vi "niFpgaMemoryEmulationRefIn.vi"(0 "Address":u32, 1 "Name":variant, 5 "Data":i32, 7 "Write? (F)":bool, 9 "inTimedLoop":bool, 11 "error in (no error)":errorcluster, 12 "Node Link":cluster{"VIRef":refnum<vi>, "UID":i32}) -> (6 "Data":i32, 15 "error out":errorcluster)   [LabVIEW 2017]
uses:
  <vilib>/rvi/DataTransferAndStorage/Container/Common/niFpgaContainerMetaDataKey.ctl
  <instcachedir>/0/nirvimemoryFastEmulation_424FDD443BC54103A00327FF1F2580B8.lvgen/nirvimemoryFastEmulation_424FDD443BC54103A00327FF1F2580B8_000.vi
  <instcachedir>/0/nirvimemoryEmulation_DE953D9D328548638838B08CDB120B27.lvgen/nirvimemoryEmulation_DE953D9D328548638838B08CDB120B27_000.vi
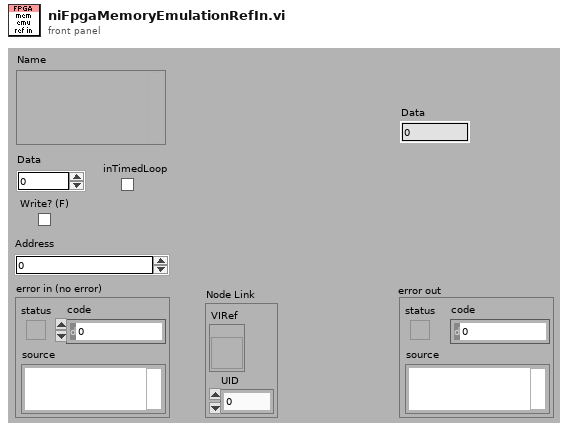
[diagram p1: front panel]
types:
  T1 = typedef "niFpgaContainerMetaDataKey.ctl" = enum16{"FPGA FIFO", "FPGA Memory", "FPGA Register", "FPGA Handshake"}
  T2 = typedef "niFpgaContainerState.ctl" = cluster{"displayName":string, "hardwareName":string, "dataType":T3, "elementTypeDescriptor":variant, "terminalTypeDescriptor":variant, "requestedNumberOfElements":u32, "memoryType":T4, "arbitrationForInterfaceA":T5, "numberOfElementsPerRead":u32, "arbitrationForInterfaceB":T5, "numberOfElementsPerWrite":u32, "VI_Defined":bool, "type":T6, "initializationParameters":T7, "disableOnOverflow/Underflow":bool, "interfaceConfiguration":T8, "controlLogic":T9, "actualNumberOfElements":u32, "dramSelection":string, "dramMaxOustandingRequests":i32, "dramIncludeByteEnables":bool, "dramGrantTime":u32, "fullEmulation":bool, "memoryInMultipleClockDomains":bool, "memoryLatency":T10}
  T3 = typedef "niFpgaDataTypeControl.ctl" = enum32{"Boolean", "I8", "I16", "I32", "I64", "U8", "U16", "U32", "U64", "FXP", "CustomControl", "SGL"}
  T4 = typedef "niFpgaContainerImplementationControl.ctl" = enum16{"Flip-Flops", "Look-Up Table", "Block Memory", "DRAM"}
  T5 = typedef "niFpgaContainerArbitrationOptionsControl.ctl" = enum16{"Always Arbitrate", "Arbitrate if Multiple Requestors Only", "Never Arbitrate"}
  T6 = typedef "niFpgaTransferTypeControl.ctl" = enum16{"Target-Scoped", "Host to Target - DMA", "Target to Host - DMA", "Peer to Peer Reader", "Peer to Peer Writer", "Bidirectional"}
  T7 = typedef "niFpgaContainerInitializationParameters.ctl" = cluster{"initialized":bool, "VI_Path":path, "initialData":variant}
  T8 = typedef "niFpgaMemoryInterfaceConfiguration.ctl" = enum16{"Read A-Write B", "Read A-Read B"}
  T9 = typedef "niFpgaFifoControlLogicControl.ctl" = enum16{"Slice Fabric", "Target Optimal", "Built-in"}
  T10 = typedef "niFpgaContainerMemoryLatencyControl.ctl" = u16
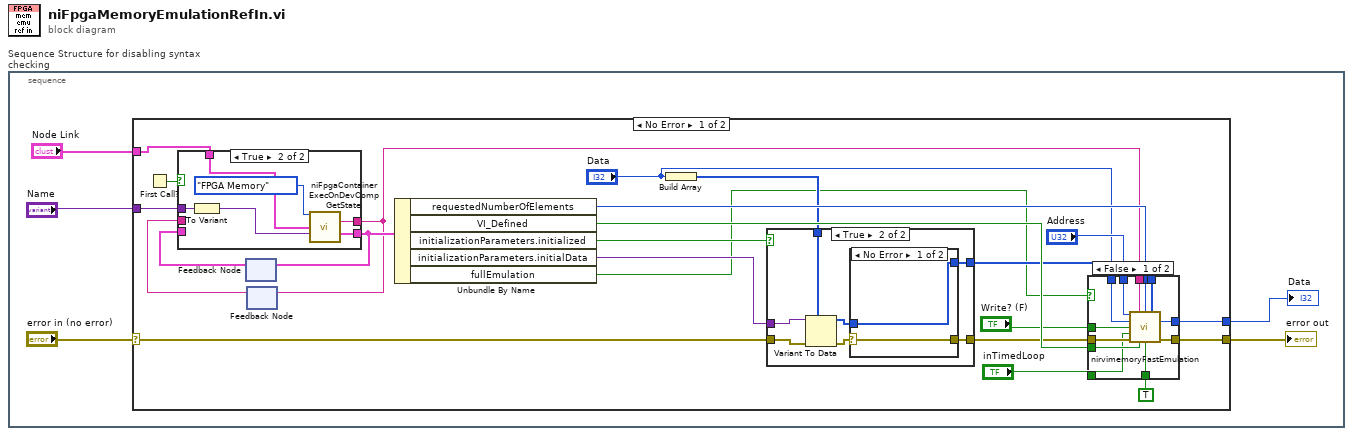
[diagram p0: block diagram]
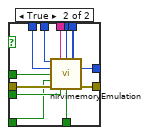
[diagram p2: hidden frame]
diagram:
  n1 = stacked-sequence "Sequence Structure for disabling syntax checking" {
    frame #0 {
      n2 = case shown="No Error" "error in (no error)" {
        selector: "error in (no error)" -> [w14 w72]
        tunnel: [w28 _] -> w3
        tunnel: [w27 w72] -> w2
        tunnel: "Name" -> [w24 _]
        tunnel: "Node Link" -> [w6 _]
        frame No Error {
          n3 = First Call?() -> (First Call?: T/F=w26:bool)
          n4 = feedback #1() -> (w17:T2)  [unwired: 1 out]
          n5 = feedback #2() -> (w15:string)  [unwired: 1 out]
          n6 = case shown="True" w26 {
            tunnel: w24 -> [_ w71]
            tunnel: [w65 w67] -> w18
            tunnel: w17 -> [w65 _]
            tunnel: [w64 w68] -> w16
            tunnel: w15 -> [w64 _]
            tunnel: w6 -> [_ w66]
            frame False {
            }
            frame True {
              n7 = To Variant(anything=w71) -> (Variant=w70:variant)
              n8 = call <vilib>:"niFpgaContainerExecOnDevCompGetState.vi"("containerMetaDataKey"=niFpgaContainerMetaDataKey."FPGA Memory", "Node Link"=w66, "name"=w70) -> ("Unique  Name"=w68:string, "containerState"=w67:T2)  [unwired: 3 in, 8 out]
            }
          }
          n9 = feedback-in #1(w18) -> ()
          n10 = feedback-in #2(w16) -> ()
          n11 = Unbundle By Name(w18) -> ("requestedNumberOfElements"=w25:u32, "VI_Defined"=w23:bool, "initializationParameters.initialized"=w8:bool, "initializationParameters.initialData"=w21:variant, "fullEmulation"=w7:bool)
          n12 = Build Array("Data") -> (w13:i32[])
          n13 = case shown="True" w8 {
            tunnel: w14 -> [w53 w59]
            tunnel: [_ w58] -> w20
            tunnel: w21 -> [_ w57]
            tunnel: [w53 w55] -> w22
            tunnel: w13 -> [_ w54]
            frame False {
            }
            frame True {
              n14 = Variant To Data(error in=w59, type=w54, Variant=w57) -> (data=w60:i32[], error out=w56:errorcluster)
              n15 = case shown="No Error" w56 {
                selector: w56 -> [w62 w63]
                tunnel: [w61 _] -> w58
                tunnel: w60 -> [w61 _]
                tunnel: [w62 w63] -> w55
                frame No Error {
                }
                frame Error {
                  # "initialized, but\nwith void value"
                }
              }
            }
          }
          n16 = case shown="False" w7 {
            tunnel: [w40 w52] -> w28
            tunnel: [w39 w51] -> w27
            tunnel: w25 -> [w38 w50]
            tunnel: w23 -> [w37 w49]
            tunnel: w22 -> [w36 w48]
            tunnel: w20 -> [w35 w47]
            tunnel: TRUE ("ref in wired") -> [w34 w46]
            tunnel: w16 -> [w33 w45]
            tunnel: "Address" -> [w32 w44]
            tunnel: "Data" -> [w31 w43]
            tunnel: "inTimedLoop" -> [w30 w42]
            tunnel: "Write? (F)" -> [w29 w41]
            frame False {
              n17 = call-generic <vilib>:"nirvimemoryFastEmulation.vi"("Address"=w32, "name"=w33, "Depth"=w38, "Initialization Data"=w35, "Data"=w31, "Write? (F)"=w29, "inTimedLoop"=w30, "error in (no error)"=w36, "Local? (F)"=w37, "ref in wired"=w34) -> ("Data"=w40:i32, "error out"=w39:errorcluster)  [unwired: 4 in]
            }
            frame True {
              n18 = call-generic <vilib>:"nirvimemoryEmulation.vi"("Address"=w44, "Name"=w45, "Depth"=w50, "Initialization Data"=w47, "Data"=w43, "Write? (F)"=w41, "inTimedLoop"=w42, "error in (no error)"=w48, "Local? (F)"=w49, "ref in wired"=w46) -> ("Data"=w52:i32, "error out"=w51:errorcluster)  [unwired: 4 in]
            }
          }
        }
        frame Error {
        }
      }
      "Data" <- w3
      "error out" <- w2
    }
  }
